vi "MainPanel.vi"() -> ()   [LabVIEW 2015]
uses:
  C:/Users/hskinner-bahay/Documents/GitHub/Kent_State_Project/Labview/LaserControl2/SlugHFVInterface/SlugHFVInterface/bin/Debug/SlugHFVInterface.dll
  SlugHFVInterface/SlugHFVInterface/bin/Debug/SlugHFVInterface.dll
  <vilib>/Instr/_visa.llb/VISA Configure Serial Port (Instr).vi
panel:
  in  "Sync Button":bool
  out "MessageQueueCnt":dbl
  in  "Pulse Spacing":u8(knob) max=60 step=10 scale=0.0..60.0
  in  "Pulse Duration":u8(knob) max=60 step=10 scale=0.0..60.0
  in  "Duty Cycle":u8(knob)=100 max=100 step=50 scale=0.0..100.0
  in  "Power Level":u8(knob)=5 max=10 step=1 scale=0.0..10.0
  out "Power On Indicator":u32(colorbox)
  out "Fault LED":bool
  in  "Stop Button 3":bool
  in  "Start Button":bool
  in  "Stop Button":bool
  in  "Load Settings Button":bool
  in  "Saved Settings Field":string(combo)
  in  "Save Settings Button":bool
  in  "Save Settings Field":string
  out "Duty Cycle Slide":i32(slide) scale=0.0..100.0
  out "Slide 2":u8(slide) scale=0.0..100.0
  in  "Load Treatment Field":string(combo)
  in  "Instructions Dialog":bool
  out "Power Level Slide":u8(slide) max=100 step=5 scale=0.0..100.0
  in  "Tab Control":T1(tab)
  out "Strength Slide":u8(slide) scale=0.0..100.0
  out "Internlock LED":bool
  out "Temperature Slide":u8(slide) scale=0.0..100.0
  out "Power On LED":bool
  out "Cooling System LED":bool
  out "RF Active LED":bool
  in  "Numeric":dbl
  in  "Numeric 2":dbl
  in  "OK Button 7":bool
  in  "OK Button 8":bool
  in  "Numeric 3":dbl
  in  "Numeric 4":dbl
  out "Numeric 5":dbl
  out "Numeric 6":dbl
  out "Numeric 7":dbl
  out "Numeric 8":dbl
  in  "String 2":string
  in  "OK Button 5":bool
  in  "HFV Interface":refnum<visa-resource-name>
  in  "HFV Interface 2":refnum<visa-resource-name>
  in  "HFV Interface 3":refnum<visa-resource-name>
  # "HFV and Laser Control Panel"
  # "Pulse Duration"
  # "Power On"
  # "Stop"
  # "Power Level"
  # "Duty Cycle"
  # "Pulse Spacing"
  # "Sync"
  # "Load Treatment"
  # "Settings"
  # "Begin Treatment"
  # "Subject Temperature"
  # "Power On"
  # "Abort"
  # "Warning"
  # "Strength"
  # "Cooling System"
  # "Interlock"
  # "RF Active"
  # "Subject Temperature"
  # "Abort Cutoff (K)"
  # "Warning Cutoff (K)"
  # "Thermo Camera"
  # "Bounding Box"
  # "Measurement Filter (K)"
  # "High"
  # "Low"
  # "Thermo Camera"
  # "Save Readings"
  # "1"
  # "Probes"
  # "2"
  # "3"
  # "HFV Port (COM)"
  # "HFV Interface Circuit (COM)"
  # "Thermo Camera"
  # "Water Chiller Status (COM)"
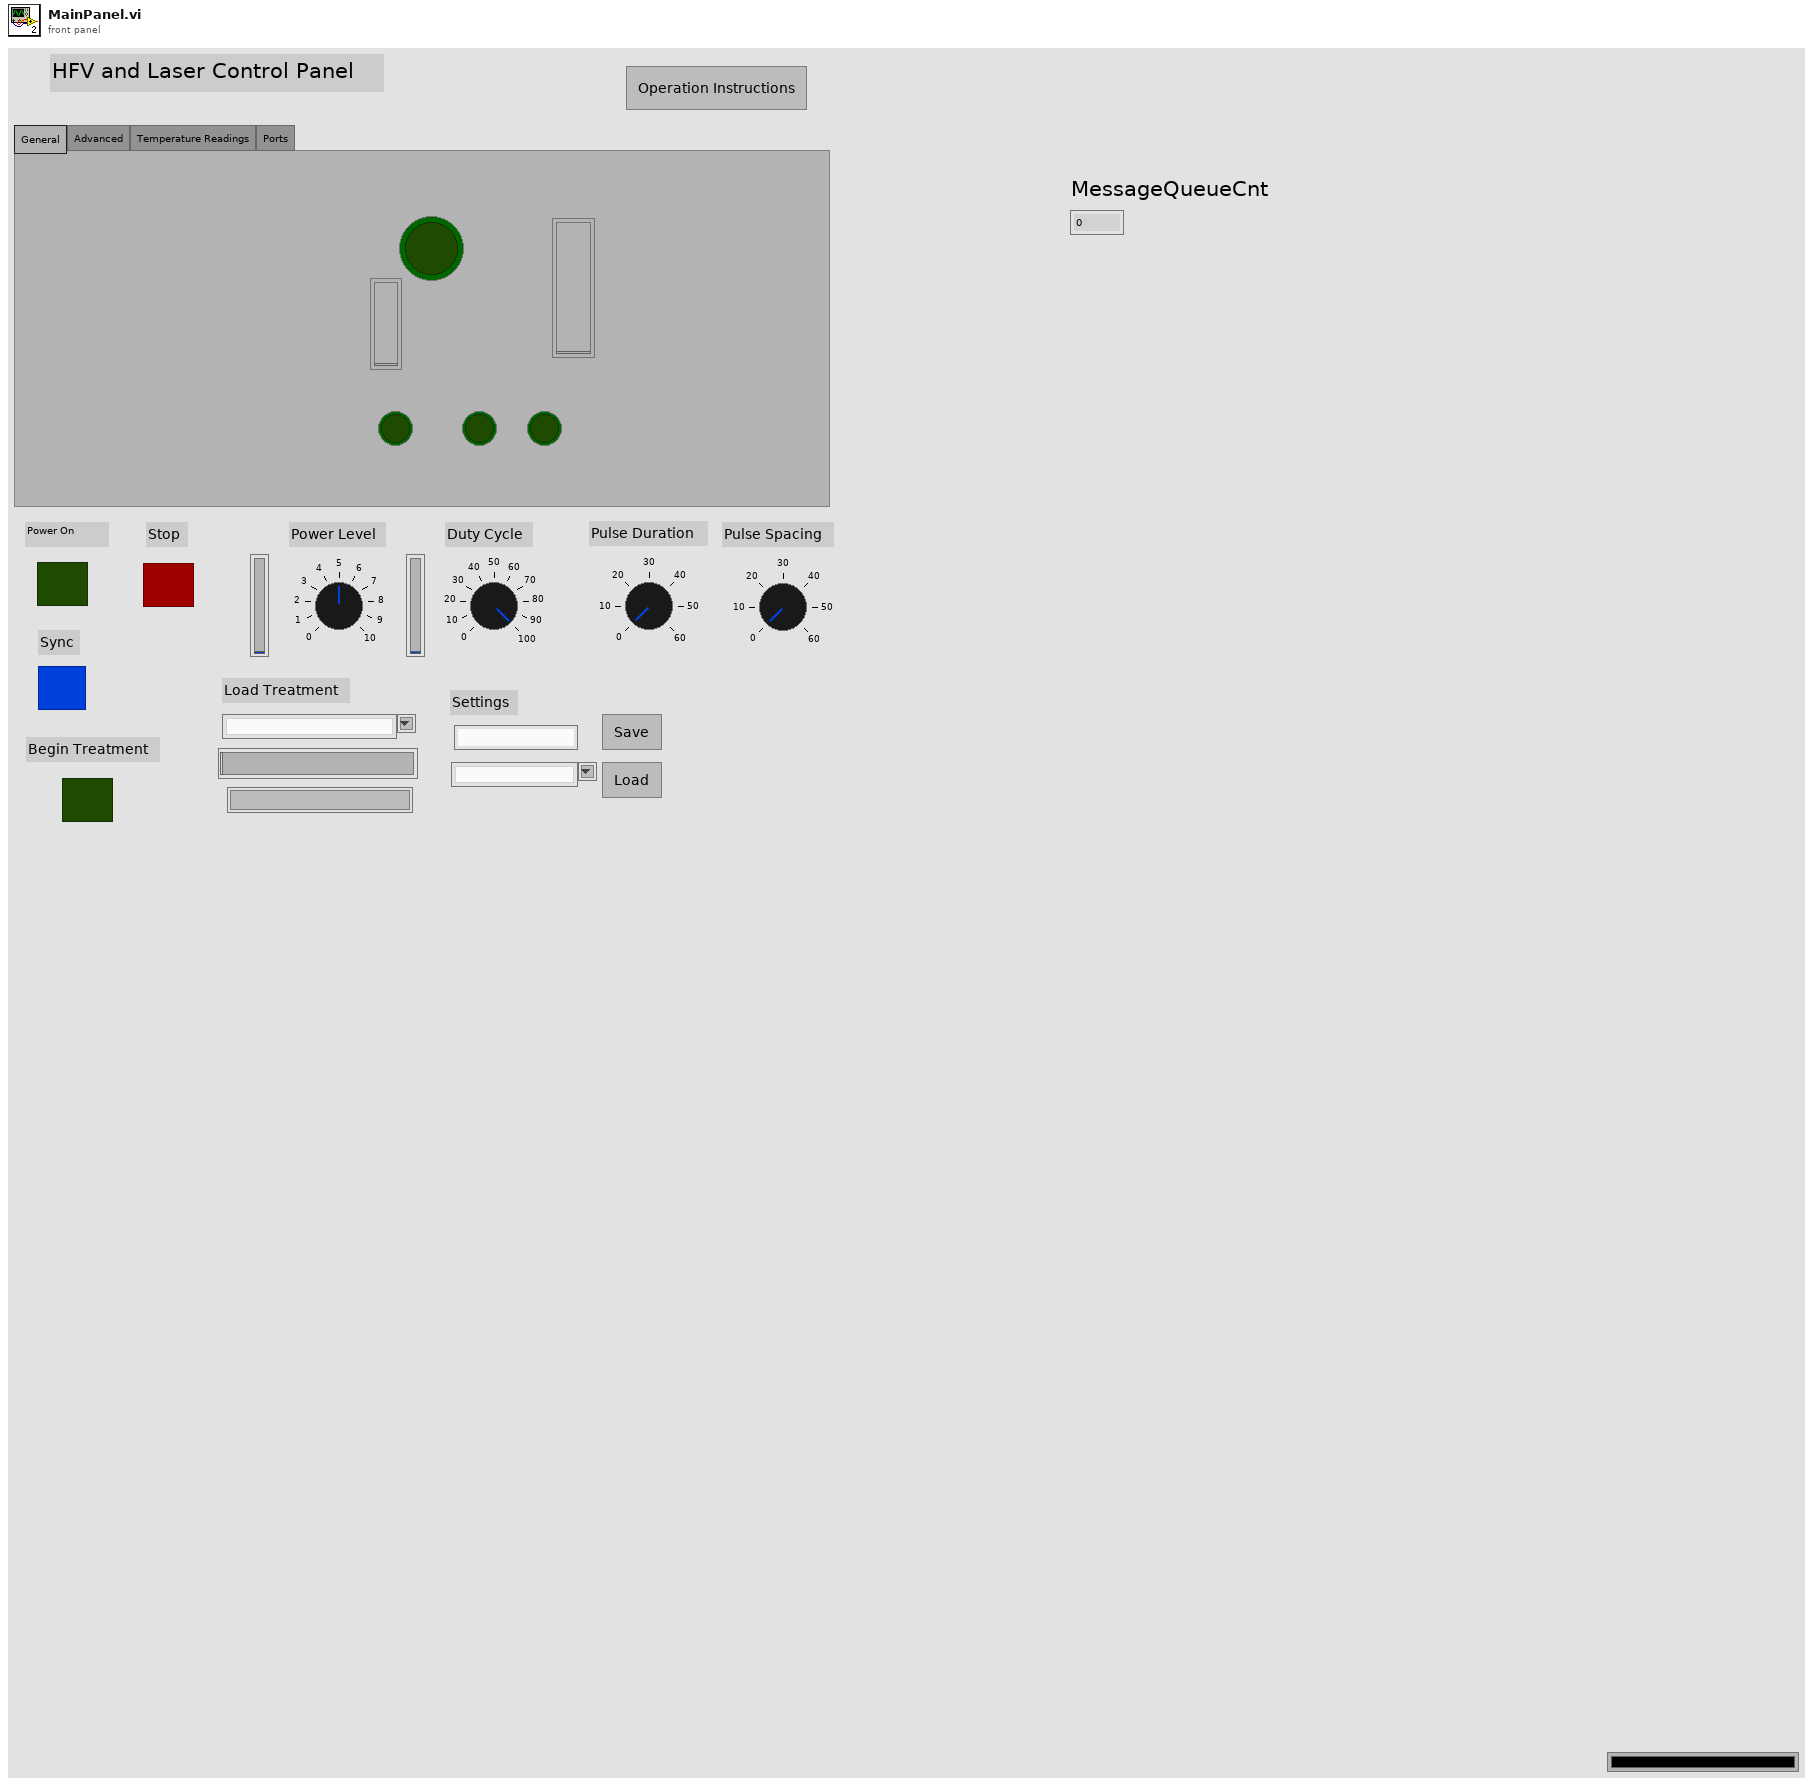
[diagram p1: front panel]
types:
  T1 = enum32{"General", "Advanced", "Temperature Readings", "Ports"}
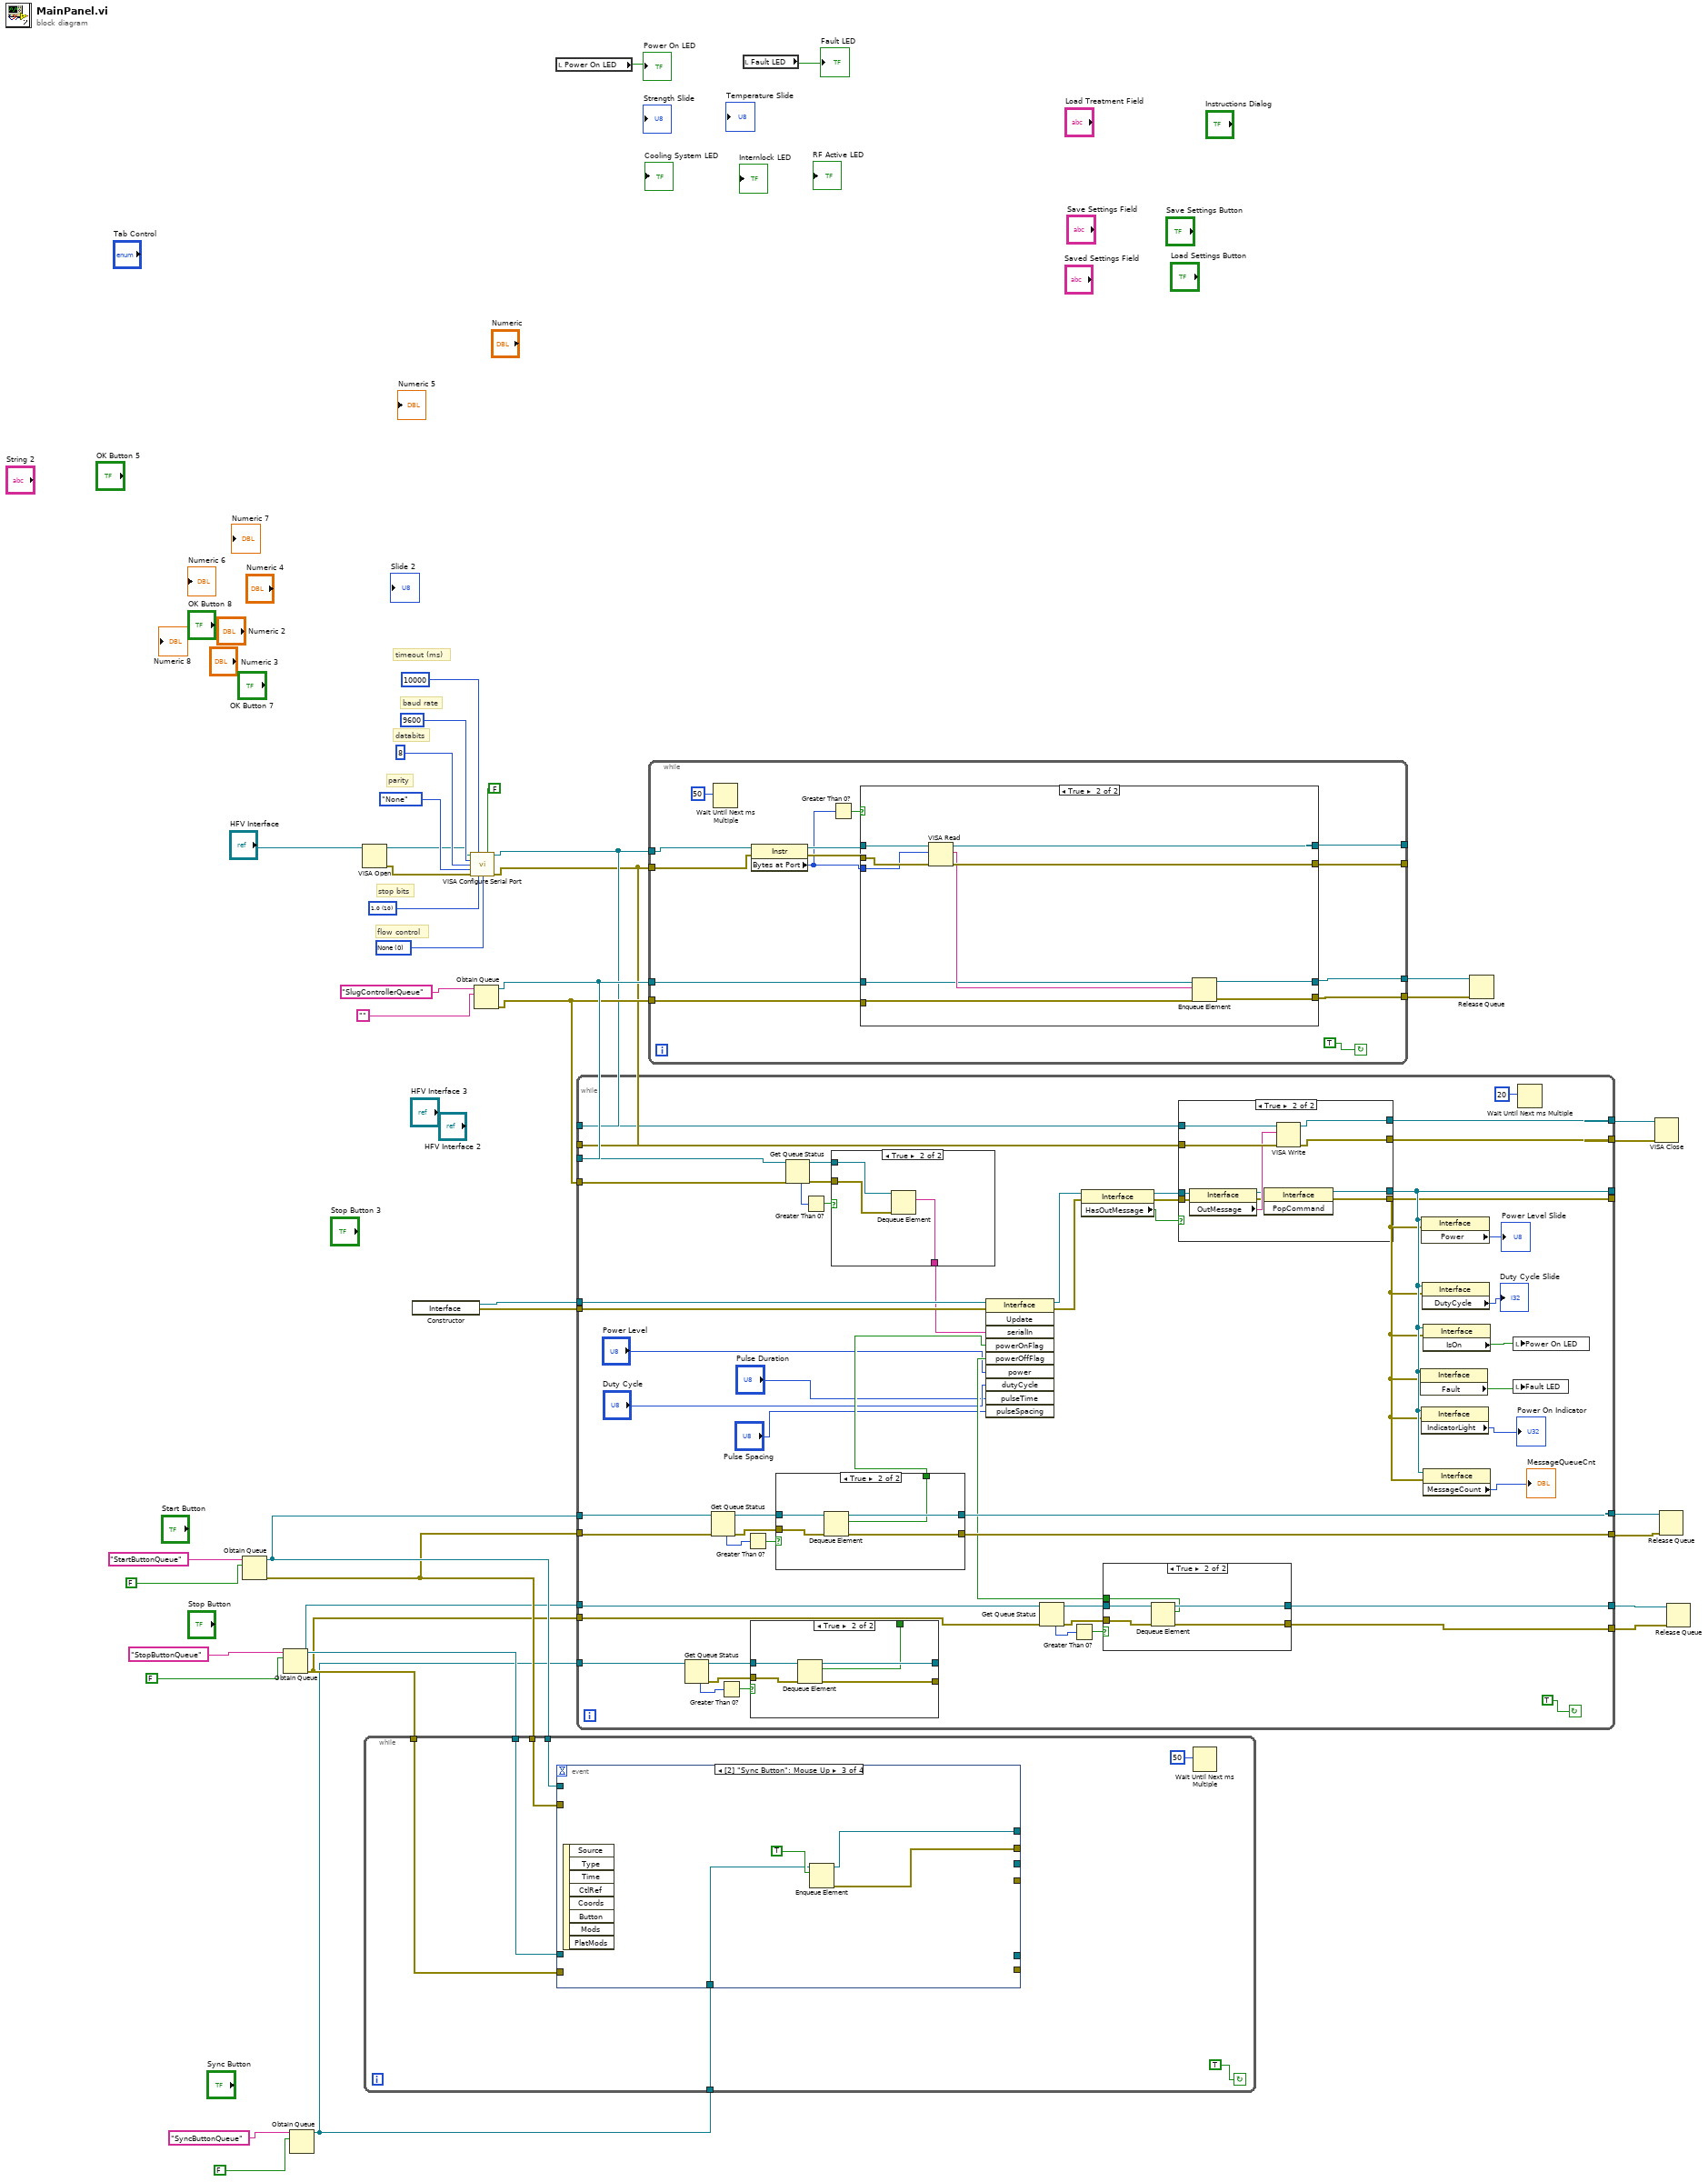
[diagram p0: block diagram]
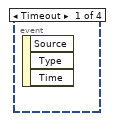
[diagram p2: hidden frame]
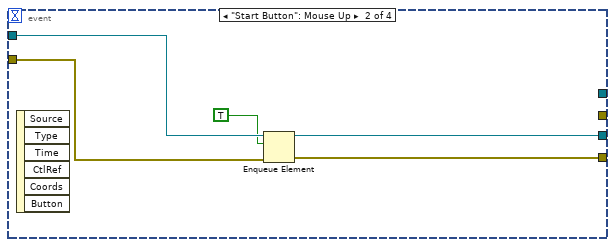
[diagram p3: hidden frame]
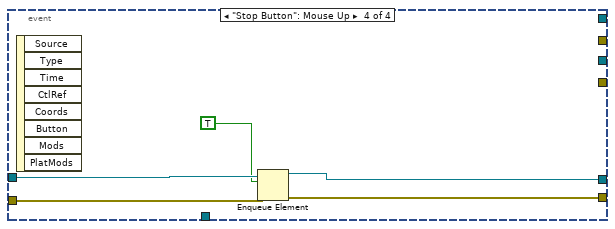
[diagram p4: hidden frame]
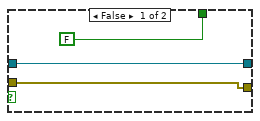
[diagram p5: hidden frame]
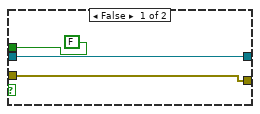
[diagram p6: hidden frame]
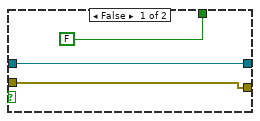
[diagram p7: hidden frame]
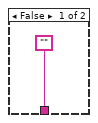
[diagram p9: hidden frame]
diagram:
  w35 = u16 0 items=["None", "XON/XOFF", "RTS/CTS", "XON/XOFF & RTS/CTS", "DTR/DSR", "XON/XOFF & DTR/DSR"] ("flow control (0:none)")
  w36 = u16 10 items=["1.0"=10, "1.5"=15, "2.0"=20] ("stop bits (10: 1 bit)")
  # "stop bits"
  # "flow control"
  # "parity"
  # "databits"
  # "baud rate"
  # "timeout (ms)"
  n1 = Obtain Queue(name (unnamed)="StartButtonQueue", element data type=FALSE) -> (queue out=w13:refnum<queue>, error out=w12:errorcluster)  [unwired: 3 in, 1 out]
  n2 = Obtain Queue(name (unnamed)="StopButtonQueue", element data type=FALSE) -> (queue out=w11:refnum<queue>, error out=w10:errorcluster)  [unwired: 3 in, 1 out]
  n3 = Obtain Queue(name (unnamed)="SyncButtonQueue", element data type=FALSE) -> (queue out=w1:refnum<queue>)  [unwired: 3 in, 2 out]
  n4 = VISA Open(VISA resource name="HFV Interface") -> (VISA resource name=w32:refnum<visa-resource-name>, error out=w31:errorcluster)  [unwired: 4 in]
  n5 = while {
    tunnel: w13 -> [w46]
    tunnel: w12 -> [w45]
    tunnel: w11 -> [w44]
    tunnel: w10 -> [w43]
    tunnel: w1 -> [w40]
    stop <- TRUE continue-if-true
    n6 = event shown="[2] \"Sync Button\": Mouse Up" {
      selector: _ -> [_ _ _ _]
      dyn-events: _ -> [_ _ _ _]
      timeout: _ -> [_ _ _ _]
      tunnel: w46 -> [_ w51 _ _]
      tunnel: [_ w50 _ _] -> _
      tunnel: [_ w49 _ _] -> _
      tunnel: w45 -> [_ w48 _ _]
      tunnel: w44 -> [_ _ _ w60]
      tunnel: w43 -> [_ _ _ w59]
      tunnel: [_ _ _ w58] -> _
      tunnel: [_ _ _ w57] -> _
      tunnel: w40 -> [_ _ w54 _]
      tunnel: [_ _ w53 _] -> _
      tunnel: [_ _ w52 _] -> _
      event Timeout {
        n7 = event-data() -> ()  [unwired: 1 in, 3 out]
      }
      event "Start Button": Mouse Up {
        n8 = event-data() -> ()  [unwired: 1 in, 6 out]
        n9 = Enqueue Element(queue=w51, element=TRUE, error in (no error)=w48) -> (queue out=w50:refnum<queue>, error out=w49:errorcluster)  [unwired: 1 in, 1 out]
      }
      event "Sync Button": Mouse Up {
        n10 = event-data() -> ()  [unwired: 1 in, 8 out]
        n11 = Enqueue Element(queue=w54, element=TRUE) -> (queue out=w53:refnum<queue>, error out=w52:errorcluster)  [unwired: 2 in, 1 out]
      }
      event "Stop Button": Mouse Up {
        n12 = event-data() -> ()  [unwired: 1 in, 8 out]
        n13 = Enqueue Element(queue=w60, element=TRUE, error in (no error)=w59) -> (queue out=w58:refnum<queue>, error out=w57:errorcluster)  [unwired: 1 in, 1 out]
      }
    }
    n14 = Wait Until Next ms Multiple(millisecond multiple=50) -> ()  [unwired: 1 out]
  }
  n15 = constructor class="Interface"() -> (reference out=w23:refnum<k24>, error out=w22:errorcluster)  [unwired: 3 in, 1 out]
  n16 = call-poly "VISA Configure Serial Port"("VISA resource name"=w32, "timeout (10sec)"=10000, "Enable Termination\nChar (T)"=FALSE ("Enable Termination\nChar (T)"), "baud rate (9600)"=9600, "data bits (8)"=8, "parity (0:none)"=enum16{"None", "Odd", "Even", "Mark", "Space"}."None", "error in (no error)"=w31, "stop bits (10: 1 bit)"=w36, "flow control (0:none)"=w35) -> ("VISA resource name out"=w21:refnum<visa-resource-name>, "error out"=w20:errorcluster)  [unwired: 5 in]
  n17 = Obtain Queue(name (unnamed)="SlugControllerQueue", element data type="") -> (queue out=w25:refnum<queue>, error out=w24:errorcluster)  [unwired: 3 in, 1 out]
  n18 = local read "Power On LED"() -> (→"Power On LED":bool)
  n19 = while {
    tunnel: w25 -> [w114]
    tunnel: w24 -> [w113]
    tunnel: w23 -> [w110]
    tunnel: w22 -> [w109]
    tunnel: w21 -> [w101]
    tunnel: w20 -> [w100]
    tunnel: [w68] -> _
    tunnel: [w67] -> _
    tunnel: [w97] -> w19
    tunnel: [w96] -> w18
    tunnel: w13 -> [w92]
    tunnel: w12 -> [w91]
    tunnel: [w88] -> w9
    tunnel: [w87] -> w8
    tunnel: w11 -> [w82]
    tunnel: w10 -> [w81]
    tunnel: [w80] -> w7
    tunnel: [w79] -> w6
    tunnel: w1 -> [w61]
    stop <- TRUE continue-if-true
    n20 = Get Queue Status(queue=w61) -> (queue out=w63:refnum<queue>, error out=w62:errorcluster, # elements in queue=w64:i32)  [unwired: 2 in, 5 out]
    n21 = Get Queue Status(queue=w92, error in (no error)=w91) -> (queue out=w90:refnum<queue>, error out=w89:errorcluster, # elements in queue=w93:i32)  [unwired: 1 in, 5 out]
    n22 = Greater Than 0?(x=w64) -> (x > 0?=w65:bool)
    n23 = Greater Than 0?(x=w93) -> (x > 0?=w94:bool)
    n24 = case shown="True" w65 {
      tunnel: w63 -> [w118 w123]
      tunnel: w62 -> [w117 w122]
      tunnel: [w118 w121] -> _
      tunnel: [w117 w120] -> _
      tunnel: [FALSE w119] -> _
      frame False {
      }
      frame True {
        n25 = Dequeue Element(queue=w123, error in (no error)=w122) -> (queue out=w121:refnum<queue>, element=w119:bool, error out=w120:errorcluster)  [unwired: 1 in, 1 out]
      }
    }
    n26 = case shown="True" w94 {
      tunnel: w90 -> [w134 w139]
      tunnel: w89 -> [w133 w138]
      tunnel: [w134 w137] -> w88
      tunnel: [w133 w136] -> w87
      tunnel: [FALSE w135] -> w77
      frame False {
      }
      frame True {
        n27 = Dequeue Element(queue=w139, error in (no error)=w138) -> (queue out=w137:refnum<queue>, element=w135:bool, error out=w136:errorcluster)  [unwired: 1 in, 1 out]
      }
    }
    n28 = Get Queue Status(queue=w114, error in (no error)=w113) -> (queue out=w107:refnum<queue>, error out=w106:errorcluster, # elements in queue=w111:i32)  [unwired: 1 in, 5 out]
    n29 = Greater Than 0?(x=w111) -> (x > 0?=w112:bool)
    n30 = case shown="True" w112 {
      tunnel: ["" w156] -> w108
      tunnel: w107 -> [_ w158]
      tunnel: w106 -> [_ w157]
      frame False {
      }
      frame True {
        n31 = Dequeue Element(queue=w158, error in (no error)=w157) -> (element=w156:string)  [unwired: 1 in, 3 out]
      }
    }
    n32 = Get Queue Status(queue=w82, error in (no error)=w81) -> (queue out=w84:refnum<queue>, error out=w83:errorcluster, # elements in queue=w85:i32)  [unwired: 1 in, 5 out]
    n33 = Greater Than 0?(x=w85) -> (x > 0?=w86:bool)
    n34 = case shown="True" w86 {
      tunnel: w84 -> [w126 w131]
      tunnel: w83 -> [w125 w130]
      tunnel: [w126 w129] -> w80
      tunnel: [w125 w128] -> w79
      tunnel: [FALSE w127] -> w78
      frame False {
      }
      frame True {
        n35 = Dequeue Element(queue=w131, error in (no error)=w130) -> (queue out=w129:refnum<queue>, element=w127:bool, error out=w128:errorcluster)  [unwired: 1 in, 1 out]
      }
    }
    n36 = invoke class="Interface" method="Update"(reference=w110, error in=w109, "serialIn"=w108, "powerOnFlag"=w77, "powerOffFlag"=w78, "power"="Power Level", "dutyCycle"="Duty Cycle", "pulseTime"="Pulse Duration", "pulseSpacing"="Pulse Spacing") -> (reference out=w104:refnum<k24>, error out=w103:errorcluster)  [unwired: 1 in, 8 out]
    n37 = property class="Interface"(reference=w104, error in=w103) -> (reference out=w99:refnum<k24>, error out=w98:errorcluster, "HasOutMessage"=w102:bool)
    n38 = case shown="True" w102 {
      tunnel: w101 -> [w141 w154]
      tunnel: w100 -> [w140 w153]
      tunnel: w99 -> [w143 w152]
      tunnel: w98 -> [w142 w151]
      tunnel: [w143 w147] -> w68
      tunnel: [w142 w146] -> w67
      tunnel: [w141 w145] -> w97
      tunnel: [w140 w144] -> w96
      frame False {
      }
      frame True {
        n39 = property class="Interface"(reference=w152, error in=w151) -> (reference out=w149:refnum<k24>, error out=w148:errorcluster, "OutMessage"=w150:string)
        n40 = invoke class="Interface" method="PopCommand"(reference=w149, error in=w148) -> (reference out=w147:refnum<k24>, error out=w146:errorcluster)  [unwired: 1 in, 1 out]
        n41 = VISA Write(VISA resource name=w154, write buffer=w150, error in (no error)=w153) -> (VISA resource name out=w145:refnum<visa-resource-name>, error out=w144:errorcluster)  [unwired: 1 out]
      }
    }
    n42 = property class="Interface"(reference=w68, error in=w67) -> ("Fault"=w76:bool)  [unwired: 2 out]
    n43 = property class="Interface"(reference=w68, error in=w67) -> ("IndicatorLight"=→"Power On Indicator":i32)  [unwired: 2 out]
    n44 = property class="Interface"(reference=w68, error in=w67) -> ("Power"=→"Power Level Slide":i32)  [unwired: 2 out]
    n45 = property class="Interface"(reference=w68, error in=w67) -> ("DutyCycle"=→"Duty Cycle Slide":i32)  [unwired: 2 out]
    n46 = property class="Interface"(reference=w68, error in=w67) -> ("IsOn"=w95:bool)  [unwired: 2 out]
    n47 = property class="Interface"(reference=w68, error in=w67) -> ("MessageCount"=→"MessageQueueCnt":i32)  [unwired: 2 out]
    n48 = local write "Power On LED"(w95) -> ()
    n49 = local write "Fault LED"(w76) -> ()
    n50 = Wait Until Next ms Multiple(millisecond multiple=20) -> ()  [unwired: 1 out]
  }
  n51 = while {
    tunnel: w21 -> [w161]
    tunnel: [w168] -> _
    tunnel: [w167] -> _
    tunnel: w25 -> [w159]
    tunnel: w24 -> [w164]
    tunnel: [w163] -> w29
    tunnel: [w162] -> w28
    tunnel: w20 -> [w160]
    stop <- TRUE continue-if-true
    n52 = Wait Until Next ms Multiple(millisecond multiple=50) -> ()  [unwired: 1 out]
    n53 = property class="Instr"(reference=w161, error in=w160) -> (reference out=w171:refnum<visa-resource-name>, error out=w172:errorcluster, "Bytes at Port"=w166:u32)
    n54 = Greater Than 0?(x=w166) -> (x > 0?=w170:bool)
    n55 = case shown="True" w170 {
      tunnel: w172 -> [w175 w186]
      tunnel: w171 -> [w176 w185]
      tunnel: [w176 w184] -> w168
      tunnel: [w175 w183] -> w167
      tunnel: w166 -> [_ w182]
      tunnel: w159 -> [w174 w180]
      tunnel: w164 -> [w173 w179]
      tunnel: [w174 w178] -> w163
      tunnel: [w173 w177] -> w162
      frame False {
      }
      frame True {
        n56 = VISA Read(VISA resource name=w185, byte count=w182, error in (no error)=w186) -> (VISA resource name out=w184:refnum<visa-resource-name>, read buffer=w181:string, error out=w183:errorcluster)  [unwired: 1 out]
        n57 = Enqueue Element(queue=w180, element=w181, error in (no error)=w179) -> (queue out=w178:refnum<queue>, error out=w177:errorcluster)  [unwired: 1 in, 1 out]
      }
    }
  }
  n58 = local read "Fault LED"() -> (→"Fault LED":bool)
  n59 = Release Queue(queue=w29, error in (no error)=w28) -> ()  [unwired: 1 in, 3 out]
  n60 = VISA Close(VISA resource name=w19, error in (no error)=w18) -> ()  [unwired: 1 out]
  n61 = Release Queue(queue=w9, error in (no error)=w8) -> ()  [unwired: 1 in, 3 out]
  n62 = Release Queue(queue=w7, error in (no error)=w6) -> ()  [unwired: 1 in, 3 out]
